vi "PI Convert 1.7 to 2.0.vi"(0 "Prompted Inputs 1.7 Test Parameters":T6={"Measurement"={"Field"="", "Value"="", "Type"=enum."Scalar", "Units"=""}, "Limit"={"Limits On"=TRUE, "Limits"=[]}}) -> (2 "Prompted Inputs 2.0 Test Parameters":T1)   [LabVIEW 2011]
uses:
  TypeDefs/PI Test Parameters v1.7.ctl
  TypeDefs/PI Test Parameters.ctl
  TypeDefs/PI Measurement Cluster.ctl
  TypeDefs/PI Limit Parameters.ctl
  TypeDefs/PI Limit Definition.ctl
  TypeDefs/PI Limit Comparison.ctl
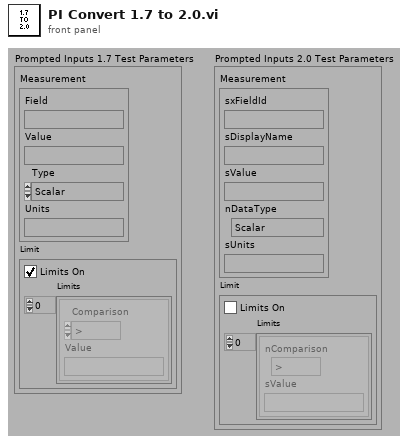
[diagram p1: front panel]
types:
  T1 = typedef "PI Test Parameters.ctl" = cluster{"Measurement":T2, "Limit":T3}
  T2 = typedef "PI Measurement Cluster.ctl" = cluster{"sxFieldId":string, "sValue":string, "nDataType":enum16{"Scalar", "Enumeration"}, "sUnits":string, "sDisplayName":string}
  T3 = typedef "PI Limit Parameters.ctl" = cluster{"Limits On":bool, "Limits":T4[]}
  T4 = typedef "PI Limit Definition.ctl" = cluster{"nComparison":T5, "sValue":string}
  T5 = typedef "PI Limit Comparison.ctl" = enum16{">", ">=", "<", "<=", "<>", "="}
  T6 = typedef "PI Test Parameters v1.7.ctl" = cluster{"Measurement":cluster{"Field":string, "Value":string, "Type":enum16{"Scalar", "Enumeration"}, "Units":string}, "Limit":cluster{"Limits On":bool, "Limits":cluster{"Comparison":enum16{">", ">=", "<", "<=", "<>", "="}, "Value":string}[]}}
  T7 = typedef "Connection Refnum.ctl" = cluster{"Environment Handle":i32, "Connection Handle":i32}
  T8 = cluster{"Comparison":enum16{">", ">=", "<", "<=", "<>", "="}, "Value":string}[]
  T9 = typedef "Field Record.ctl" = cluster{"ixField":i32, "iSequenceOrder":i32, "sxFieldId":string, "sxSequenceId":string, "sDisplayName":string, "sValue":string, "sUnits":string, "nDataType":T10, "nNextItem":T11, "fSystem":bool, "fSystemValue":bool, "fRequired":bool, "fSetAtTest":bool, "fTestField":bool, "fDeleted":bool, "fIndexed":bool, "fFreeList":bool}
  T10 = typedef "Field DataTypes.ctl" = enum32{"text", "numeric", "list", "timestamp", "boolean"}
  T11 = typedef "Field NextItem.ctl" = enum32{"Reset", "Retain", "Auto-Increment"}
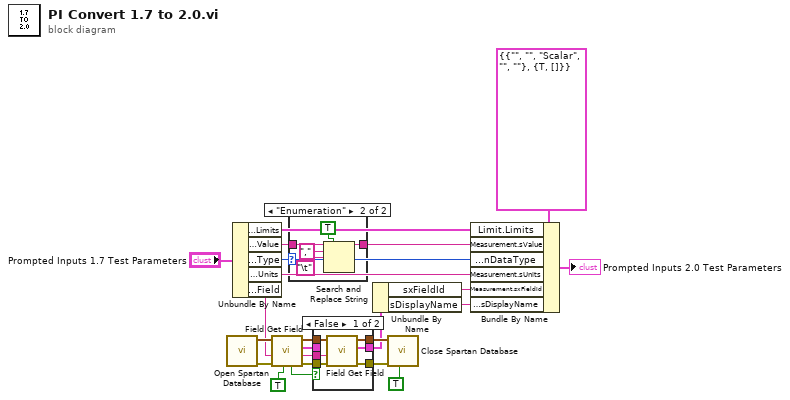
[diagram p0: block diagram]
diagram:
  n1 = call "Open Spartan Database.vi"() -> ("error out"=w17:errorcluster, "Connection Refnum"=w16:T7)  [unwired: 10 in]
  n2 = Unbundle By Name("Prompted Inputs 1.7 Test Parameters") -> ("Limit.Limits"=w19:T8, "Measurement.Value"=w4:string, "Measurement.Type"=w2:enum16{"Scalar", "Enumeration"}, "Measurement.Units"=w18:string, "Measurement.Field"=w5:string)
  n3 = call "Field Get Field.vi"("by sDisplayName? (f, by sFieldId)"=TRUE, "error in (no error)"=w17, "sFieldId or sDisplayName (\"\")"=w5, "Connection Refnum"=w16) -> ("error out"=w13:errorcluster, "Field"=w11:T9, "Connection Refnum"=w12:T7, "Data Present?"=w14:bool)  [unwired: 1 in, 3 out]
  n4 = case shown="\"Enumeration\"" w2 {
    tunnel: w4 -> [w23 w28]
    tunnel: [w23 w27] -> w3
    frame "Scalar" {
    }
    frame "Enumeration" {
      n5 = Search and Replace String(replace all?=TRUE ("replace all? (F)"), input string=w28, search string=",", replace string="\t") -> (result string=w27:string)  [unwired: 1 in, 6 out]
    }
  }
  n6 = case shown="False" w14 {
    tunnel: w13 -> [w34 w35]
    tunnel: w12 -> [w33 w36]
    tunnel: w11 -> [_ w37]
    tunnel: [w32 w37] -> w8
    tunnel: [w31 w36] -> w10
    tunnel: [w30 w35] -> w9
    tunnel: w5 -> [w29 _]
    frame False {
      n7 = call "Field Get Field.vi"("error in (no error)"=w34, "sFieldId or sDisplayName (\"\")"=w29, "Connection Refnum"=w33) -> ("error out"=w30:errorcluster, "Field"=w32:T9, "Connection Refnum"=w31:T7)  [unwired: 2 in, 4 out]
    }
    frame True {
    }
  }
  n8 = Unbundle By Name(w8) -> ("sxFieldId"=w7:string, "sDisplayName"=w6:string)
  n9 = call "Close Spartan Database.vi"("Force Close? (f)"=TRUE ("by sDisplayName? (f, by sFieldId)"), "error in (no error)"=w9, "Connection Refnum"=w10) -> ()  [unwired: 8 in, 1 out]
  n10 = Bundle By Name(cluster=T1 {"Measurement"={"sxFieldId"="", "sValue"="", "nDataType"=enum."Scalar", "sUnits"="", "sDisplayName"=""}, "Limit"={"Limits On"=TRUE, "Limits"=[]}} ("Prompted Inputs Test Parameters"), "Limit.Limits"=w19, "Measurement.sValue"=w3, "Measurement.nDataType"=w2, "Measurement.sUnits"=w18, "Measurement.sxFieldId"=w7, "Measurement.sDisplayName"=w6) -> (→"Prompted Inputs 2.0 Test Parameters":T1)
